vi "update globals from exec.vi"(1 "Manual Temp control":bool, 2 "Manual Power":dbl, 3 "Setpoint (C)":dbl=30.0, 11 "PID exp exec":T2, 12 "exec.T mode":T1) -> (4 "T params":T4={"Setpoint"=30.0, "Control Bandwidth"=4.0, "Integral Time"=30.0, "Int\nON"=TRUE, "Derivative Tme"=0.5, "Der\nON"=TRUE, "Settle Bandwidth"=1.0, "Settle Time"=30.0} {"Settle Time" step=1.0; "Settle Bandwidth" step=0.01; "Derivative Tme" step=0.01; "Integral Time" step=1.0; "Control Bandwidth" step=0.1; "Setpoint" step=0.1}, 8 "Total elapsed time (s)":dbl=30.0, 15 "PID exp exec out":T2)   [LabVIEW 2019]
doc: "This subVI updates the bug global variables from the executive thread.\n\nPaul K Dixon\nP3600\nCSUSB Physics"
uses:
  typedefs/temp cont cluster.ctl
  typedefs/temp exec cluster.ctl
  typedefs/temp mode enum.ctl
  typedefs/temp indicator.ctl
  typedefs/temp control status.ctl
  typedefs/PID control parameters.ctl
  typedefs/temp cont utility.ctl
  typedefs/PID exec cluster.ctl
  typedefs/bug temp file info.ctl
  globals/Bug temp globals.vi
panel:
  out "T cont out":T5 {"utility"."therm volt" format="%_6g"; "utility"."heat volt in" format="%_6g"; "utility"."heat volt out" format="%_6g"; "utility"."power out" format="%_6g"; "utility"."H Vmax" format="%_6g"; "exec"."man power" format="%_6g"; "exec"."exec setpoint" format="%_6g"; "T params"."Settle Time" step=1.0; "T params"."Settle Bandwidth" step=0.01; "T params"."Derivative Tme" step=0.01; "T params"."Integral Time" step=1.0; "T params"."Control Bandwidth" step=0.1; "T params"."Setpoint" step=0.1; "T status"."Setpoint" format="%_6g"; "T status"."Power" format="%_6g"; "T status"."Temp" format="%_6g"}
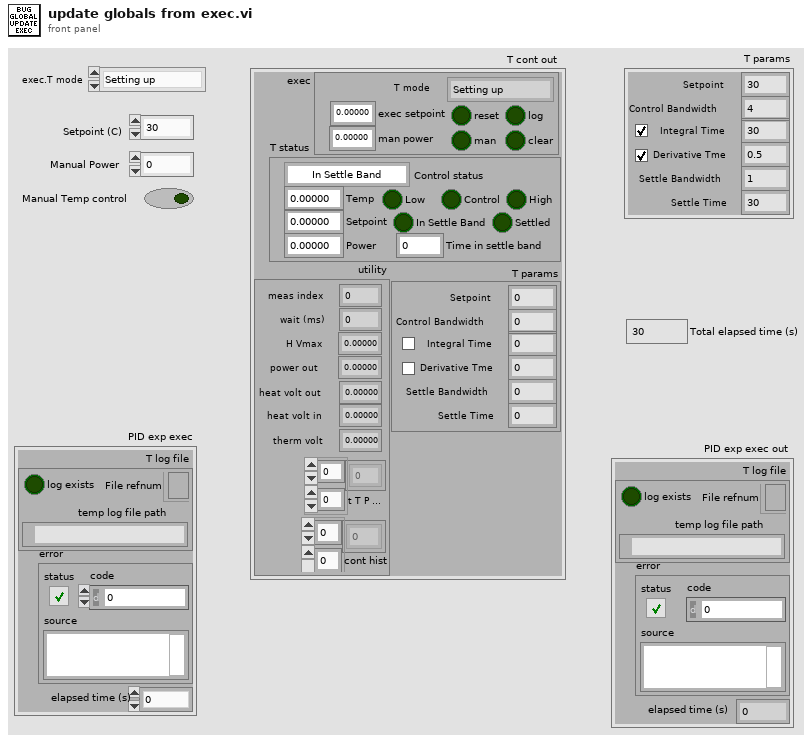
[diagram p1: front panel]
types:
  T1 = typedef "temp mode enum.ctl" = enum16{"Setting up", "Listening to exec", "Exit"}
  T2 = typedef "PID exec cluster.ctl" = cluster{"T log file":T3, "error":errorcluster, "elapsed time (s)":dbl}
  T3 = typedef "bug temp file info.ctl" = cluster{"log exists":bool, "File refnum":refnum<file>, "temp log file path":path}
  T4 = typedef "PID control parameters.ctl" = cluster{"Setpoint":dbl, "Control Bandwidth":dbl, "Integral Time":dbl, "Int\nON":bool, "Derivative Tme":dbl, "Der\nON":bool, "Settle Bandwidth":dbl, "Settle Time":dbl}
  T5 = typedef "temp cont cluster.ctl" = cluster{"exec":T6, "T status":T7, "T params":T4, "utility":T9}
  T6 = typedef "temp exec cluster.ctl" = cluster{"T mode":T1, "exec setpoint":dbl, "reset":bool, "man power":dbl, "man":bool, "log":bool, "clear":bool}
  T7 = typedef "temp indicator.ctl" = cluster{"Control status":T8, "Temp":dbl, "Power":dbl, "Time in settle band":dbl, "Settled":bool, "Low":bool, "High":bool, "Setpoint":dbl, "Control":bool, "In Settle Band":bool}
  T8 = typedef "temp control status.ctl" = enum16{"In Settle Band", "In Control Band", "Below Control Band", "Above Control Band"}
  T9 = typedef "temp cont utility.ctl" = cluster{"meas index":i32, "wait (ms)":i32, "H Vmax":dbl, "power out":dbl, "heat volt out":dbl, "heat volt in":dbl, "therm volt":dbl, "t T P hist":dbl[][], "cont hist":dbl[][]}
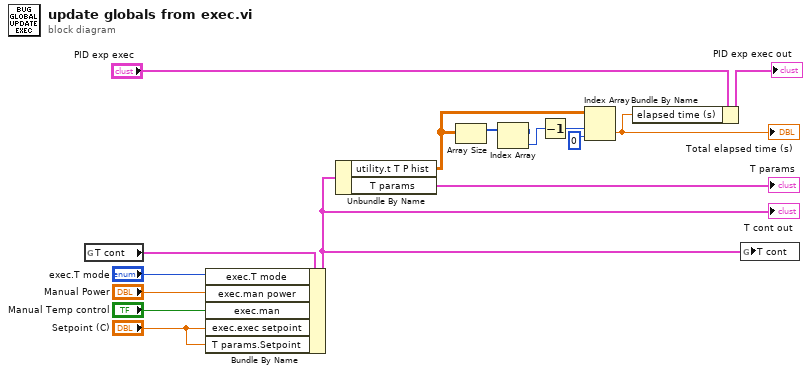
[diagram p0: block diagram]
diagram:
  n1 = global read "Bug temp globals.vi" "T cont"() -> (w12:T5)
  n2 = Bundle By Name(cluster=w12, "exec.T mode"="exec.T mode", "exec.man power"="Manual Power", "exec.man"="Manual Temp control", "exec.exec setpoint"="Setpoint (C)", "T params.Setpoint"="Setpoint (C)") -> (w11:T5)
  "T cont out" <- w11
  n3 = Unbundle By Name(w11) -> ("utility.t T P hist"=w7:dbl[][], "T params"=→"T params":T4)
  n4 = Array Size(array=w7) -> (size(s)=w4:i32[])
  n5 = Index Array(array=w4) -> (element=w3:i32)  [unwired: 1 in]
  n6 = Decrement(x=w3) -> (x-1=w5:i32)
  n7 = Index Array(array=w7, index (row)=w5, index (col)=0 ("disabled index (col)")) -> (element=w1:dbl)
  "Total elapsed time (s)" <- w1
  n8 = Bundle By Name(cluster="PID exp exec", "elapsed time (s)"=w1) -> (→"PID exp exec out":T2)
  n9 = global write "Bug temp globals.vi" "T cont"(w11) -> ()
